vi "GetSampleValues.vi"() -> (2 "input":cluster{"x":dbl[], "y":dbl[], "z":dbl[]})   [LabVIEW 2014]
uses:
  <vilib>/myRIO/Instrument Drivers/Onboard IO/DIO/typedefs/DIO Reference.ctl
  <vilib>/myRIO/Common/Instrument Driver Framework/Utilities/typedefs/myRIO Generic Hardware Reference.ctl
  <vilib>/myRIO/Common/Instrument Driver Framework/Utilities/typedefs/Hardware Version Enum.ctl
  <vilib>/myRIO/Common/Instrument Driver Framework/Utilities/typedefs/myRIO v1.0 Reference.ctl
  <vilib>/myRIO/Common/Instrument Driver Framework/Utilities/typedefs/Generic FPGA Reference.ctl
  <vilib>/myRIO/Common/Instrument Driver Framework/myRIO v1.0/DIO/typedefs/DIO Channels List.ctl
  <vilib>/myRIO/Common/Instrument Driver Framework/myRIO v1.0/DIO/typedefs/DIO Channels Enum.ctl
  <vilib>/userdefined/High Color/nirio_resource_hc.ctl
  <vilib>/myRIO/Common/Instrument Driver Framework/Utilities/vis/Is FPGA Ref Available.vi
  <vilib>/myRIO/Common/Instrument Driver Framework/myRIO v1.0/DIO/vis/myRIO v1.1 Open DIO.vi
  <vilib>/myRIO/Instrument Drivers/Onboard IO/DIO/vis/Read.vi
  <vilib>/myRIO/Common/Instrument Driver Framework/Utilities/vis/Validate Channels.vi
  <vilib>/myRIO/Common/Instrument Driver Framework/myRIO v1.0/DIO/vis/myRIO v1.0 Reserve DIO.vi
  <vilib>/myRIO/Common/Instrument Driver Framework/myRIO v1.0/Resource Manager/vis/myRIO v1.0 Reserve Channel List.vi
  <vilib>/myRIO/Common/Instrument Driver Framework/myRIO v1.0/DIO/vis/myRIO v1.0 Build MUX Configuration DIO.vi
  <vilib>/myRIO/Common/Instrument Driver Framework/myRIO v1.0/Resource Manager/vis/myRIO v1.0 Reserve Channel.vi
  <vilib>/myRIO/Common/Instrument Driver Framework/myRIO v1.0/Resource Manager/vis/myRIO v1.0 Unreserve Channel.vi
  <vilib>/myRIO/Common/Instrument Driver Framework/myRIO v1.0/Resource Manager/vis/myRIO v1.0 Create Configuration List.vi
  <vilib>/myRIO/Common/Instrument Driver Framework/myRIO v1.0/Resource Manager/vis/myRIO v1.0 Build Mutex Name.vi
  <vilib>/Utility/VariantDataType/GetNumericInfo.vi
  <vilib>/Utility/error.llb/Error Cluster From Error Code.vi
  <vilib>/myRIO/Common/Instrument Driver Framework/myRIO v1.0/myRIO v1.1 Open.vi
  <vilib>/myRIO/Common/Instrument Driver Framework/Utilities/vis/IO Manager.vi
  <vilib>/myRIO/Common/Instrument Driver Framework/Utilities/vis/Configuration Manager.vi
  <vilib>/myRIO/Common/Instrument Driver Framework/myRIO v1.0/Resource Manager/vis/myRIO v1.0 Configure IO.vi
  <vilib>/myRIO/Common/Instrument Driver Framework/myRIO v1.0/myRIO v1.0 Close.vi
  <vilib>/myRIO/Common/Instrument Driver Framework/myRIO v1.0/DIO/vis/myRIO v1.0 Read DIO.vi
  <vilib>/myRIO/Express VI/Onboard Devices/Button/Button Express VI.xnode
  <vilib>/myRIO/Instrument Drivers/Onboard IO/DIO/vis/myRIO DIO Open.xnode
  <vilib>/myRIO/Instrument Drivers/Onboard IO/DIO/DIO.lvlib
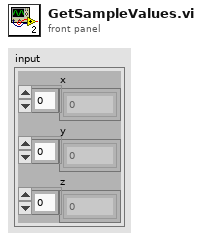
[diagram p1: front panel]
types:
  T1 = enum16{"Learn X", "Learn Y", "Learn Z", "Done Learning"}
  T2 = typedef "DIO.lvlib/DIO Reference.ctl" = cluster{"myRIO Reference":T3, "DIO Channels List":T7}
  T3 = typedef "myRIO Generic Hardware Reference.ctl" = cluster{"myRIO Model":T4, "myRIO Hardware Reference":T5}
  T4 = typedef "Hardware Version Enum.ctl" = enum16{"Unknown", "myRIO-1900", "myRIO-1950"}
  T5 = typedef "myRIO v1.0 Reference.ctl" = cluster{"Generic FPGA Reference":T6, "Allow multiple opens":bool}
  T6 = typedef "Generic FPGA Reference.ctl" = refnum<k20>
  T7 = typedef "DIO Channels List.ctl" = T8[]
  T8 = typedef "DIO Channels Enum.ctl" = enum16{"Not Connected", "C/DIO0", "C/DIO1", "C/DIO2", "C/DIO3", "C/DIO4", "C/DIO5", "C/DIO6", "C/DIO7", "A/DIO0", "A/DIO1", "A/DIO2", "A/DIO3", "A/DIO4", "A/DIO5", "A/DIO6", "A/DIO7", "A/DIO8", "A/DIO9", "A/DIO10", "A/DIO11", "A/DIO12", "A/DIO13", "A/DIO14", "A/DIO15", "B/DIO0", "B/DIO1", "B/DIO2", "B/DIO3", "B/DIO4", "B/DIO5", "B/DIO6", "B/DIO7", "B/DIO8", "B/DIO9", "B/DIO10", "B/DIO11", "B/DIO12", "B/DIO13", "B/DIO14", "B/DIO15", "LED0", "LED1", "LED2", "LED3", "Button0"}
  T9 = typedef "nirio_resource_hc.ctl" = tag
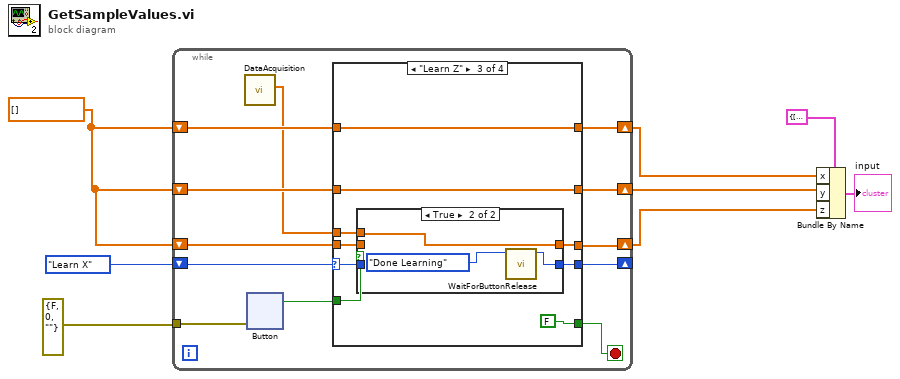
[diagram p0: block diagram]
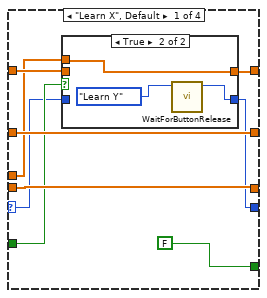
[diagram p2: hidden frame]
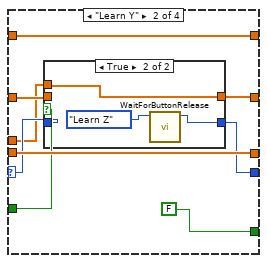
[diagram p4: hidden frame]
diagram:
  w6 = dbl[] [] ("x train 2")
  n1 = while {
    tunnel: errorcluster {"status"=FALSE, "code"=0, "source"=""} ("error constant") -> [w13]
    shift-right: [w17] -> w5
    shift-left: w6 -> [w18]
    shift-right: [w15] -> w4
    shift-left: w6 -> [w16]
    shift-right: [w11] -> w3
    shift-left: w6 -> [w12]
    shift-right: [w9] -> _
    shift-left: T1."Learn X" -> [w20]
    stop <- w19 stop-if-true
    n2 = call "DataAcquisition.vi"() -> ("appended array"=w10:dbl[])  [unwired: 10 in, 1 out]
    n3 = xnode "Button"("error in (no error)"=w13) -> ("Value"=w14:bool)  [unwired: 1 out]
    n4 = case shown="\"Learn Z\"" w20 {
      selector: w20 -> [w57 w72 w85 w98]
      tunnel: [FALSE FALSE FALSE w102] -> w19
      tunnel: w14 -> [w58 w73 w86 w102]
      tunnel: [w60 w77 w91 w101] -> w17
      tunnel: w18 -> [w61 w77 w91 w101]
      tunnel: w16 -> [w63 w75 w90 w100]
      tunnel: [w63 w74 w90 w100] -> w15
      tunnel: w12 -> [w62 w76 w89 w99]
      tunnel: [w62 w76 w88 w99] -> w11
      tunnel: w10 -> [w59 w70 w87 _]
      tunnel: [w56 w71 w84 w98] -> w9
      frame "Learn X", Default {
        n5 = case shown="True" w58 {
          tunnel: w61 -> [w66 _]
          tunnel: [w66 w69] -> w60
          tunnel: w59 -> [_ w69]
          tunnel: w57 -> [w65 _]
          tunnel: [w65 w67] -> w56
          frame False {
          }
          frame True {
            n6 = call "WaitForButtonRelease.vi"("Enum in"=T1."Learn Y") -> ("Enum out"=w67:T1)  [unwired: 10 in]
          }
        }
      }
      frame "Learn Y" {
        n7 = case shown="True" w73 {
          tunnel: w75 -> [w80 _]
          tunnel: [w80 w83] -> w74
          tunnel: w70 -> [_ w83]
          tunnel: w72 -> [w79 _]
          tunnel: [w79 w81] -> w71
          frame False {
          }
          frame True {
            n8 = call "WaitForButtonRelease.vi"("Enum in"=T1."Learn Z") -> ("Enum out"=w81:T1)  [unwired: 10 in]
          }
        }
      }
      frame "Learn Z" {
        n9 = case shown="True" w86 {
          tunnel: w89 -> [w94 _]
          tunnel: [w94 w97] -> w88
          tunnel: w87 -> [_ w97]
          tunnel: w85 -> [w93 _]
          tunnel: [w93 w96] -> w84
          frame False {
          }
          frame True {
            n10 = call "WaitForButtonRelease.vi"("Enum in"=T1."Done Learning") -> ("Enum out"=w96:T1)  [unwired: 10 in]
          }
        }
      }
      frame "Done Learning" {
      }
    }
  }
  n11 = Bundle By Name(cluster=cluster{"x":dbl[], "y":dbl[], "z":dbl[]} {"x"=[], "y"=[], "z"=[]}, "x"=w5, "y"=w4, "z"=w3) -> (→"input":cluster{"x":dbl[], "y":dbl[], "z":dbl[]})
